vi "get processed data (XYplot).vi"(8 "error in (no error)":errorcluster, 11 "Task in":refnum<class "Task.lvclass">) -> (0 "error out":errorcluster, 2 "Processed data (XY plot)":cluster{dbl[], dbl[]}[](graph), 3 "Task out":refnum<class "Task.lvclass">)   [LabVIEW 2020, in "Tasks.lvlib" / "Task.lvclass"]
uses:
  Task.lvclass
  Task.lvclass/Task.ctl
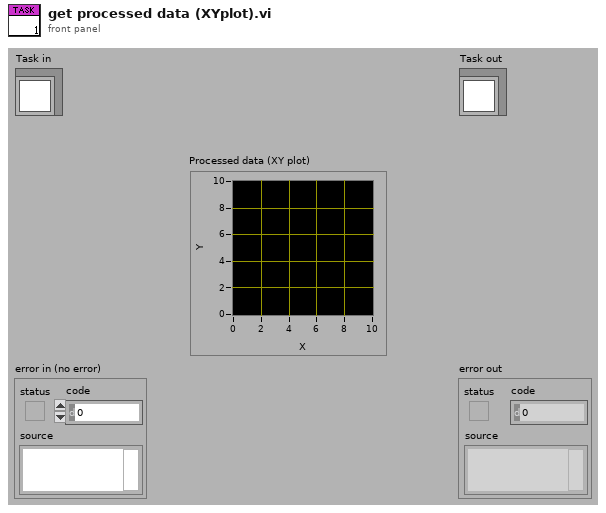
[diagram p1: front panel]
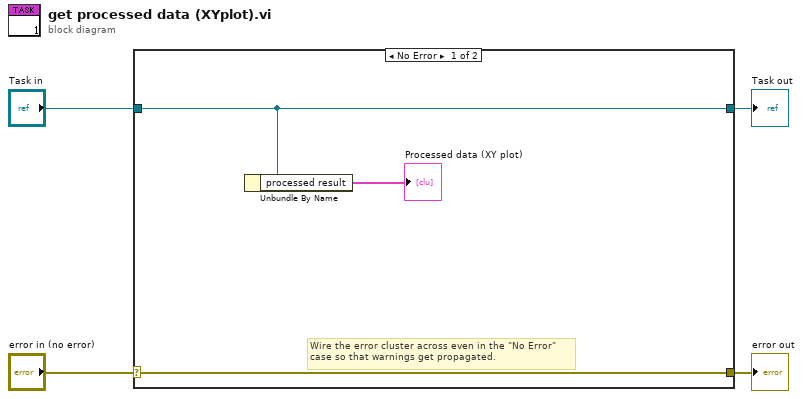
[diagram p0: block diagram]
diagram:
  n1 = case shown="No Error" "error in (no error)" {
    selector: "error in (no error)" -> [w7 w9]
    tunnel: [w7 w9] -> w3
    tunnel: [w6 w8] -> w1
    tunnel: "Task in" -> [w6 w8]
    frame No Error {
      # "Wire the error cluster across even in the \"No Error\"\ncase so that warnings get propagated."
      n2 = Unbundle By Name(w6) -> ("processed result"=→"Processed data (XY plot)":cluster{dbl[], dbl[]}[])
    }
    frame Error {
    }
  }
  "error out" <- w3
  "Task out" <- w1
